vi "Init.vi"(8 "error in":errorcluster, 11 "Custom Events in":refnum<class "Custom Events.lvclass">) -> (0 "error out":errorcluster, 3 "Custom Events out":refnum<class "Custom Events.lvclass">)   [LabVIEW 2024, in "SourceGrid.lvlib" / "Custom Events.lvclass"]
uses:
  Custom Events.lvclass
  Custom Events.lvclass/Custom Events.ctl
  D:/git/Sourcegrid-LabVIEW/dll/SourceGrid.dll
  dll/SourceGrid.dll
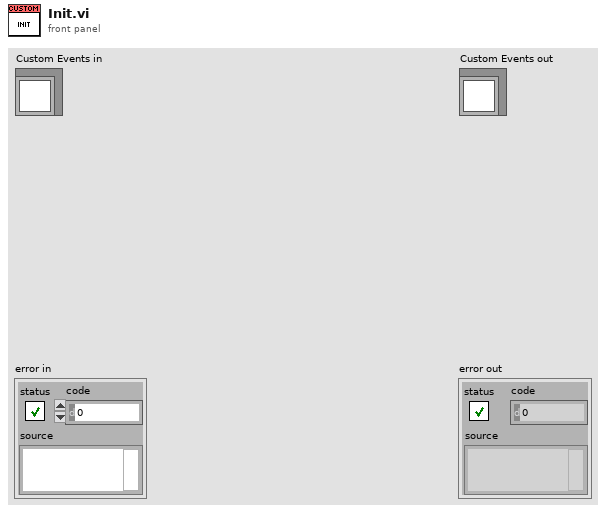
[diagram p1: front panel]
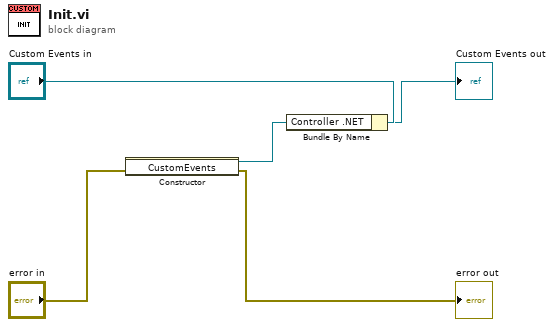
[diagram p0: block diagram]
diagram:
  n1 = constructor class="CustomEvents"(error in="error in") -> (reference out=w2:refnum<k24>, error out=→"error out":errorcluster)  [unwired: 2 in, 1 out]
  n2 = Bundle By Name(cluster="Custom Events in", "Controller .NET"=w2) -> (→"Custom Events out":refnum<class "Custom Events.lvclass">)
